vi "FMA1600A General Setup.vi"(5 "Gas Type":T4, 7 "Unit ID":string, 8 "error in (no error)":errorcluster, 9 "Select Gas?":bool=TRUE, 10 "Set STP Register":bool, 11 "VISA Refnum in":refnum<visa-resource-name>) -> (0 "error out":errorcluster, 1 "Data Frame Format":T1, 2 "Measurement Units":T2, 3 "VISA Refnum out":refnum<visa-resource-name>)   [LabVIEW 2020]
uses:
  Type Definitions/FMA1600A Gas Type.ctl
  Type Definitions/FMA1600A Units String.ctl
  Units of Measure.ctl
  Data Frame.ctl
  Type Definitions/FMA1600A Commands.ctl
  <vilib>/Utility/error.llb/whitespace.ctl
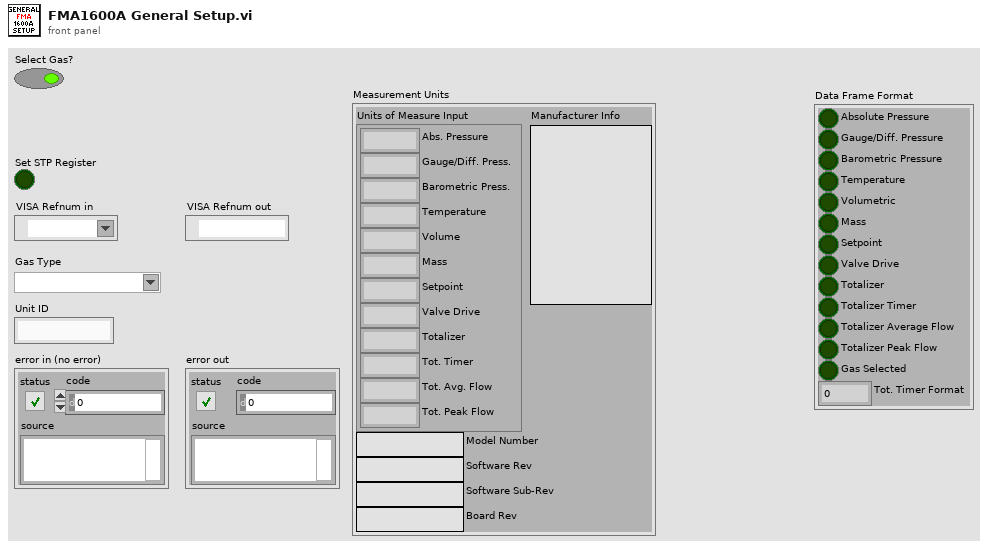
[diagram p1: front panel]
types:
  T1 = typedef "Data Frame.ctl" = cluster{"Absolute Pressure":bool, "Gauge/Diff. Pressure":bool, "Barometric Pressure":bool, "Temperature":bool, "Volumetric":bool, "Mass":bool, "Setpoint":bool, "Valve Drive":bool, "Totalizer":bool, "Totalizer Timer":bool, "Totalizer Average Flow":bool, "Totalizer Peak Flow":bool, "Gas Selected":bool, "Tot. Timer Format":u16}
  T2 = typedef "FMA1600A Units String.ctl" = cluster{"Software Rev":string, "Model Number":string, "Manufacturer Info":string, "Software Sub-Rev":string, "Board Rev":string, "Units of Measure Input":T3}
  T3 = typedef "Units of Measure.ctl" = cluster{"Abs. Pressure":string, "Gauge/Diff. Press.":string, "Barometric Press.":string, "Temperature":string, "Volume":string, "Mass":string, "Setpoint":string, "Valve Drive":string, "Totalizer":string, "Tot. Timer":string, "Tot. Avg. Flow":string, "Tot. Peak Flow":string}
  T4 = typedef "FMA1600A Gas Type.ctl" = string
  T5 = enum8{"2400", "9600", "19200", "38400", "57600", "115200", "Unknown"}
  T6 = cluster{"Valve Drive":bool, "Totalizer":bool, "Totalizer Timer":bool, "Totalizer Peak Flow":bool, "Show Abs., Gauge\nand Baro. pressures":bool}
  T7 = cluster{"Pressure(s)":bool, "Temperature":bool, "Volumetric":bool, "Mass":bool, "Totalizer Average Flow":bool, "Gas Selected":bool}
  T8 = typedef "whitespace.ctl" = u16
  T9 = typedef "FMA1600A Commands.ctl" = string
  T10 = cluster{"Unit ID":string, "Baud Rate":enum8{"2400", "9600", "19200", "38400", "57600", "115200", "Unknown"}, "VISA Sesssion In":refnum<visa-resource-name>}
  T11 = cluster{"Abs. Pressure":string, "Gauge/Diff. Press.":string, "Barometric Press.":string, "Temperature":string, "Volume":string, "Mass":string, "Setpoint":string, "Valve Drive":string, "Totalizer":string, "Tot. Timer":string, "Tot. Avg. Flow":string, "Tot. Peak Flow":string}
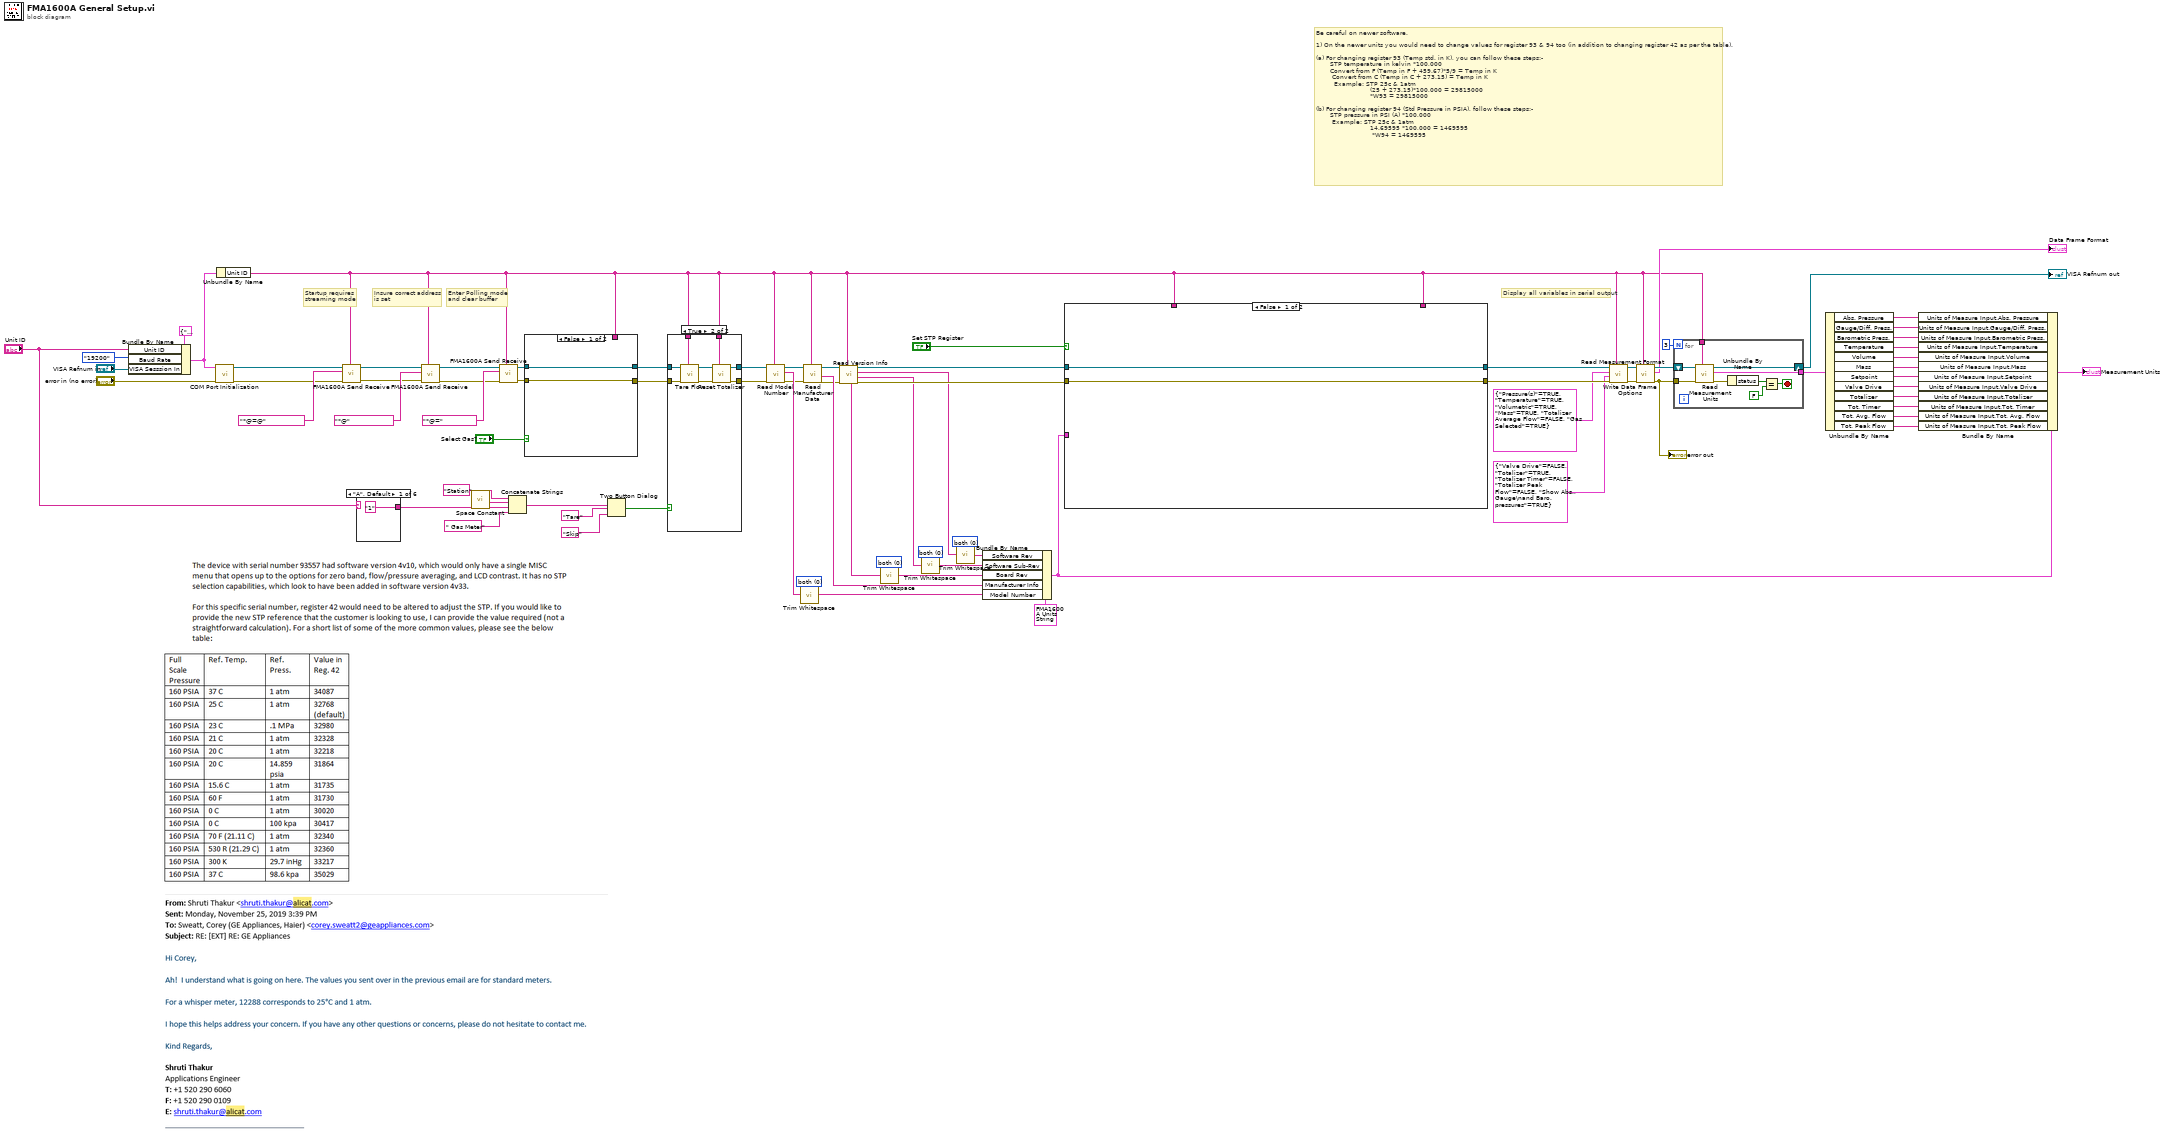
[diagram p0: block diagram]
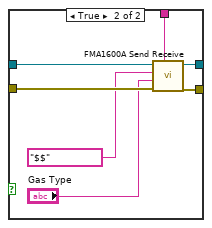
[diagram p2: hidden frame]
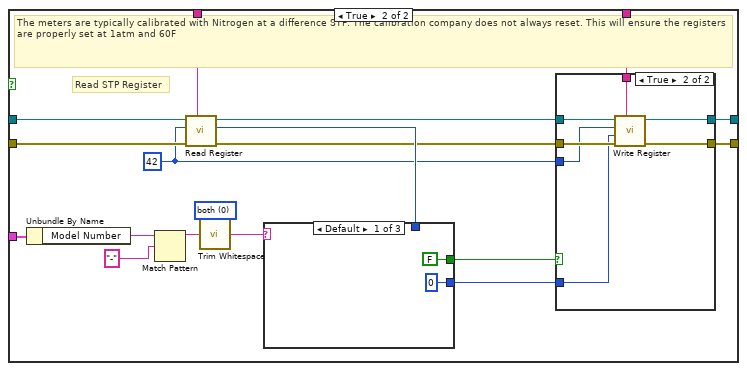
[diagram p3: hidden frame]
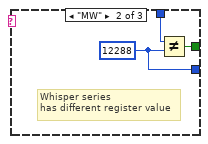
[diagram p5: hidden frame]
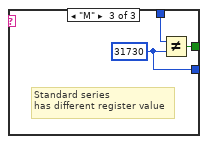
[diagram p6: hidden frame]
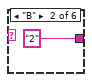
[diagram p7: hidden frame]
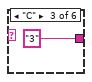
[diagram p8: hidden frame]
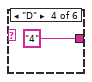
[diagram p9: hidden frame]
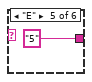
[diagram p10: hidden frame]
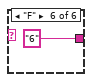
[diagram p11: hidden frame]
diagram:
  w17 = T8 0 items=["both", "start of string", "end of string"] ("location (both)")
  w18 = T8 0 items=["both", "start of string", "end of string"] ("location (both)")
  w21 = T8 0 items=["both", "start of string", "end of string"] ("location (both)")
  w22 = T8 0 items=["both", "start of string", "end of string"] ("location (both)")
  # "Display all variables in serial output"
  # "Enter Polling mode\nand clear buffer"
  # "Startup requires \nstreaming mode"
  # "Insure correct address\nis set"
  # "Be careful on newer software.\n\n1) On the newer units you would need to change values for register 93 & 94 too (in addition to changing register 42 as per the table). \n\n(a) For changing register 93 (Temp std. in K), you can follow these steps:-\n       STP temperature in kelvin *100,000\n       Convert from F (Temp in F + 459.67)*5/9 = Temp in K\n        Convert from C (Temp in C + 273.15) = Temp in K\n         Example: STP 25c & 1atm\n                           (25 + 273.15)*100,000 = 29815000\n                           *W93 = 29815000\n\n(b) For changing register 94 (Std Pressure in PSIA), follow these steps:-\n       STP pressure in PSI (A) *100,000\n        Example: STP 25c & 1atm\n                           14.69595 *100,000 = 1469595\n                            *W94 = 1469595"
  n1 = Bundle By Name(cluster=T10 {"Unit ID"="A", "Baud Rate"=enum."19200", "VISA Sesssion In"="COM1"} ("Communication Settings"), "Unit ID"="Unit ID", "Baud Rate"=T5."19200", "VISA Sesssion In"="VISA Refnum in") -> (w62:T10)
  n2 = call "COM Port Initialization.vi"("error in (no error)"="error in (no error)", "Communication Settings"=w62) -> ("error out"=w59:errorcluster, "VISA Session Out"=w58:refnum<visa-resource-name>)  [unwired: 8 in]
  n3 = Unbundle By Name(w62) -> ("Unit ID"=w8:string)
  n4 = call "FMA1600A Send Receive.vi"("Unit ID"=w8, "error in (no error)"=w59, "FMA1600A Commands"=T9 "*@=@", "VISA Refnum in"=w58) -> ("error out"=w57:errorcluster, "VISA Refnum out"=w56:refnum<visa-resource-name>)  [unwired: 5 in, 1 out]
  n5 = case shown="\"A\", Default" "Unit ID" {
    tunnel: ["1" ("message") "2" ("message") "3" ("message") "4" ("message") "5" ("message") "6" ("message")] -> w76
    frame "A", Default {
    }
    frame "B" {
    }
    frame "C" {
    }
    frame "D" {
    }
    frame "E" {
    }
    frame "F" {
    }
  }
  n6 = call "FMA1600A Send Receive.vi"("Unit ID"=w8, "error in (no error)"=w57, "FMA1600A Commands"=T9 "*@", "VISA Refnum in"=w56) -> ("error out"=w51:errorcluster, "VISA Refnum out"=w52:refnum<visa-resource-name>)  [unwired: 5 in, 1 out]
  n7 = call <vilib>:"Space Constant.vi"() -> ("String"=w70:string)
  n8 = call "FMA1600A Send Receive.vi"("Unit ID"=w8, "error in (no error)"=w51, "FMA1600A Commands"=T9 "*@=", "VISA Refnum in"=w52) -> ("error out"=w55:errorcluster, "VISA Refnum out"=w54:refnum<visa-resource-name>)  [unwired: 5 in, 1 out]
  n9 = Concatenate Strings("Station" ("message"), w70, w76, " Gas Meter" ("string")) -> (w73:string)
  n10 = case shown="False" "Select Gas?" {
    tunnel: w55 -> [w86 w93]
    tunnel: w54 -> [w85 w92]
    tunnel: [w85 w89] -> w50
    tunnel: [w86 w88] -> w49
    tunnel: w8 -> [_ w87]
    frame False {
    }
    frame True {
      n11 = call "FMA1600A Send Receive.vi"("Unit ID"=w87, "error in (no error)"=w93, "Gas Type"="Gas Type", "FMA1600A Commands"=T9 "$$", "VISA Refnum in"=w92) -> ("error out"=w88:errorcluster, "VISA Refnum out"=w89:refnum<visa-resource-name>)  [unwired: 4 in, 1 out]
    }
  }
  n12 = Two Button Dialog(message=w73, 1:"Skip" ("F button name (\"Cancel\")"), 2:"Tare" ("T button name (\"OK\")")) -> (T button?=w78:bool)
  n13 = case shown="True" w78 {
    tunnel: [w94 w96] -> w33
    tunnel: [w95 w97] -> w34
    tunnel: w49 -> [w95 w102]
    tunnel: w50 -> [w94 w101]
    tunnel: w8 -> [_ w103]
    tunnel: w8 -> [_ w98]
    frame False {
    }
    frame True {
      n14 = call "Tare Flow.vi"("Unit ID (A)"=w103, "error in"=w102, "VISA Session In"=w101) -> ("error out"=w100:errorcluster, "VISA Session Out"=w99:refnum<visa-resource-name>)  [unwired: 7 in]
      n15 = call "Reset Totalizer.vi"("Unit ID (A)"=w98, "error in"=w100, "VISA Session In"=w99) -> ("error out"=w97:errorcluster, "VISA Session Out"=w96:refnum<visa-resource-name>)  [unwired: 6 in, 1 out]
    }
  }
  n16 = call "Read Model Number.vi"("Unit ID (A)"=w8, "error in"=w34, "VISA Session In"=w33) -> ("error out"=w4:errorcluster, "Model Number"=w24:string, "VISA Session Out"=w3:refnum<visa-resource-name>)  [unwired: 6 in]
  n17 = call <vilib>:"Trim Whitespace.vi"("string"=w24, "location (both)"=w22) -> ("trimmed string"=w23:string)
  n18 = call "Read Manufacturer Data.vi"("Unit ID (A)"=w8, "error in"=w4, "VISA Session In"=w3) -> ("error out"=w1:errorcluster, "Manufacturer Info"=w29:string, "VISA Session Out"=w2:refnum<visa-resource-name>)  [unwired: 6 in]
  n19 = call "Read Version Info.vi"("Unit ID (A)"=w8, "error in"=w1, "VISA Session In"=w2) -> ("error out"=w32:errorcluster, "Software Sub-Rev"=w16:string, "Software Rev"=w20:string, "VISA Session Out"=w31:refnum<visa-resource-name>, "Board Rev"=w14:string)  [unwired: 4 in]
  n20 = call <vilib>:"Trim Whitespace.vi"("string"=w14, "location (both)"=w18) -> ("trimmed string"=w13:string)
  n21 = call <vilib>:"Trim Whitespace.vi"("string"=w16, "location (both)"=w17) -> ("trimmed string"=w15:string)
  n22 = call <vilib>:"Trim Whitespace.vi"("string"=w20, "location (both)"=w21) -> ("trimmed string"=w19:string)
  n23 = Bundle By Name(cluster=T2 {"Software Rev"="", "Model Number"="", "Manufacturer Info"="", "Software Sub-Rev"="", "Board Rev"="", "Units of Measure Input"={"Abs. Pressure"="", "Gauge/Diff. Press."="", "Barometric Press."="", "Temperature"="", "Volume"="", "Mass"="", "Setpoint"="", "Valve Drive"="", "Totalizer"="", "Tot. Timer"="", "Tot. Avg. Flow"="", "Tot. Peak Flow"=""}} ("Measurement Units"), "Software Rev"=w19, "Software Sub-Rev"=w15, "Board Rev"=w13, "Manufacturer Info"=w29, "Model Number"=w23) -> (w28:T2)
  n24 = case shown="False" "Set STP Register" {
    tunnel: [w104 w110] -> w10
    tunnel: [w105 w113] -> w12
    tunnel: w32 -> [w105 w122]
    tunnel: w31 -> [w104 w123]
    tunnel: w8 -> [_ w106]
    tunnel: w8 -> [_ w112]
    tunnel: w28 -> [_ w121]
    frame False {
    }
    frame True {
      w117 = T8 0 items=["both", "start of string", "end of string"] ("location (both)")
      w109 = u16 42 ("Register address")
      # "Read STP Register"
      # "The meters are typically calibrated with Nitrogen at a difference STP. The calibration company does not always reset. This will ensure the registers are properly set at 1atm and 60F"
      n25 = Unbundle By Name(w121) -> ("Model Number"=w120:string)
      n26 = Match Pattern(string=w120, regular expression="-" ("search string")) -> (before substring=w118:string)  [unwired: 1 in, 3 out]
      n27 = call "Read Register.vi"("Unit ID (A)"=w106, "error in"=w122, "Register address"=w109, "VISA Session In"=w123) -> ("error out"=w114:errorcluster, "Register Value (I32)"=w115:i32, "VISA Session Out"=w111:refnum<visa-resource-name>)  [unwired: 5 in]
      n28 = call <vilib>:"Trim Whitespace.vi"("string"=w118, "location (both)"=w117) -> ("trimmed string"=w116:string)
      n29 = case shown="Default" w116 {
        tunnel: w115 -> [_ w137 w140]
        tunnel: [FALSE w136 w139] -> w107
        tunnel: [0 ("y") w135 w138] -> w108
        frame Default {
        }
        frame "MW" {
          w135 = 12288 ("y")
          # "Whisper series\nhas different register value"
          n30 = Not Equal?(x=w137, y=w135) -> (x != y?=w136:bool)
        }
        frame "M" {
          w138 = 31730 ("y")
          # "Standard series\nhas different register value"
          n31 = Not Equal?(x=w140, y=w138) -> (x != y?=w139:bool)
        }
      }
      n32 = case shown="True" w107 {
        tunnel: w114 -> [w125 w132]
        tunnel: [w125 w131] -> w113
        tunnel: w112 -> [_ w130]
        tunnel: w111 -> [w124 w129]
        tunnel: [w124 w128] -> w110
        tunnel: w109 -> [_ w127]
        tunnel: w108 -> [_ w126]
        frame False {
        }
        frame True {
          n33 = call "Write Register.vi"("Unit ID (A)"=w130, "error in"=w132, "Register Value"=w126, "Register address"=w127, "VISA Session In"=w129) -> ("error out"=w131:errorcluster, "VISA Session Out"=w128:refnum<visa-resource-name>)  [unwired: 4 in, 1 out]
        }
      }
    }
  }
  n34 = call "Write Data Frame Options.vi"("Unit ID (A)"=w8, "error in"=w12, "Enables: Data frame only"=T6 {"Valve Drive"=FALSE, "Totalizer"=TRUE, "Totalizer Timer"=FALSE, "Totalizer Peak Flow"=FALSE, "Show Abs., Gauge\nand Baro. pressures"=TRUE}, "Enables: \nData frame and Display"=T7 {"Pressure(s)"=TRUE, "Temperature"=TRUE, "Volumetric"=TRUE, "Mass"=TRUE, "Totalizer Average Flow"=FALSE, "Gas Selected"=TRUE} ("Enables: \nData frame and Display"), "VISA Session In"=w10) -> ("error out"=w11:errorcluster, "VISA Session Out"=w9:refnum<visa-resource-name>)  [unwired: 5 in]
  n35 = call "Read Measurement Format.vi"("Unit ID (A)"=w8, "error in"=w11, "VISA Session In"=w9) -> ("error out"=w25:errorcluster, "Data Frame Format"=→"Data Frame Format":T1, "VISA Session Out"=w27:refnum<visa-resource-name>)  [unwired: 6 in]
  "error out" <- w25
  n36 = for {
    N: 3 -> [_]
    tunnel: w8 -> [w143]
    tunnel: [w145] -> w48
    shift-right: [w146] -> w69
    shift-left: w27 -> [w147]
    tunnel: w25 -> [w144]
    stop <- w148 stop-if-true
    n37 = call "Read Measurement Units.vi"("Unit ID (A)"=w143, "error in"=w144, "VISA Session In"=w147) -> ("error out"=w149:errorcluster, "Measurement Units"=w145:T11, "VISA Session Out"=w146:refnum<visa-resource-name>)  [unwired: 5 in, 1 out]
    n38 = Unbundle By Name(w149) -> ("status"=w142:bool)
    n39 = Equal?(x=w142, y=FALSE ("x")) -> (x = y?=w148:bool)
  }
  "VISA Refnum out" <- w69
  n40 = Unbundle By Name(w48) -> ("Abs. Pressure"=w46:string, "Gauge/Diff. Press."=w45:string, "Barometric Press."=w44:string, "Temperature"=w43:string, "Volume"=w42:string, "Mass"=w41:string, "Setpoint"=w40:string, "Valve Drive"=w39:string, "Totalizer"=w38:string, "Tot. Timer"=w37:string, "Tot. Avg. Flow"=w36:string, "Tot. Peak Flow"=w35:string)
  n41 = Bundle By Name(cluster=w28, "Units of Measure Input.Abs. Pressure"=w46, "Units of Measure Input.Gauge/Diff. Press."=w45, "Units of Measure Input.Barometric Press."=w44, "Units of Measure Input.Temperature"=w43, "Units of Measure Input.Volume"=w42, "Units of Measure Input.Mass"=w41, "Units of Measure Input.Setpoint"=w40, "Units of Measure Input.Valve Drive"=w39, "Units of Measure Input.Totalizer"=w38, "Units of Measure Input.Tot. Timer"=w37, "Units of Measure Input.Tot. Avg. Flow"=w36, "Units of Measure Input.Tot. Peak Flow"=w35) -> (→"Measurement Units":T2)
